vi "Detect Tags.vi"(8 "error in (no error)":errorcluster, 10 "Greyscale Image":refnum<data-value>, 11 "AprilTagDetector":refnum<data-value>) -> (0 "error out":errorcluster, 2 "Detections":T1[](array[typedef]), 3 "AprilTagDetector (Duplicate)":refnum<data-value>)   [LabVIEW 2020, in "g_ar_toolkit.feature_detection.lvlib" / "AprilTagDetector.lvclass"]
uses:
  AprilTagDetector.lvclass
  Detection.ctl
  g_ar_toolkit.common/Image Point (Float).ctl
  g_ar_toolkit.common/Square Corners.ctl
  AprilTagDetector.lvclass/AprilTagDetector.ctl
  bin/g_ar_toolkit.1.32.dll
  g_ar_toolkit.common/g_ar_toolkit.common.lvlib
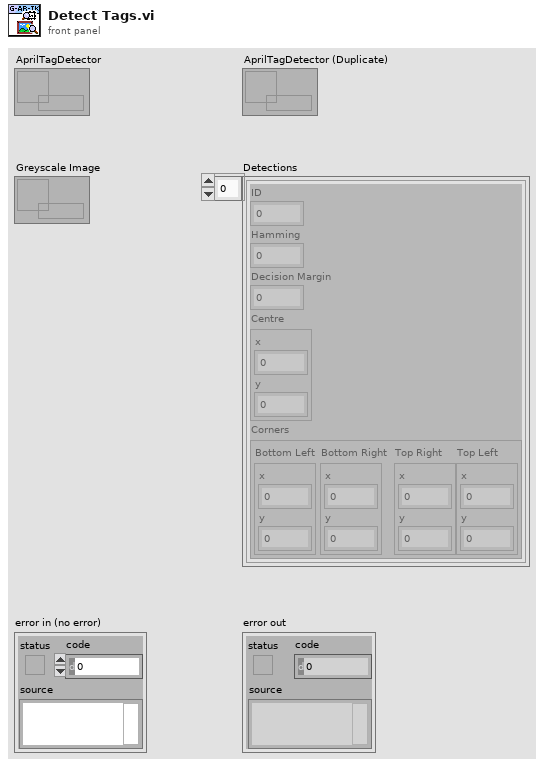
[diagram p1: front panel]
types:
  T1 = typedef "g_ar_toolkit.feature_detection.lvlib/AprilTagDetector.lvclass/Detection.ctl" = cluster{"ID":i32, "Hamming":i32, "Decision Margin":sgl, "Centre":T2, "Corners":T3}
  T2 = typedef "g_ar_toolkit.common.lvlib/Image Point (Float).ctl" = cluster{"x":dbl, "y":dbl}
  T3 = typedef "g_ar_toolkit.common.lvlib/Square Corners.ctl" = cluster{"Bottom Left":T2, "Bottom Right":T2, "Top Right":T2, "Top Left":T2}
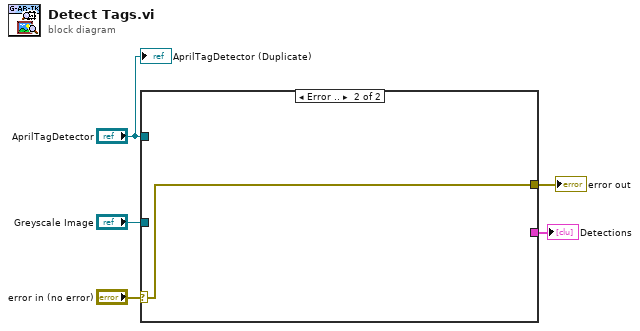
[diagram p0: block diagram]
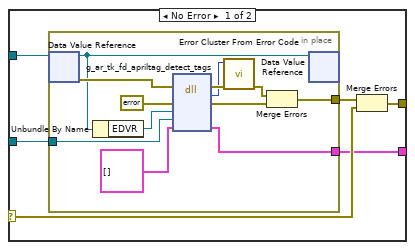
[diagram p2: hidden frame]
diagram:
  n1 = case shown="Error .." "error in (no error)" {
    selector: "error in (no error)" -> [w9 w24]
    tunnel: "Greyscale Image" -> [w11 _]
    tunnel: [w8 w24] -> w3
    tunnel: "AprilTagDetector" -> [w7 _]
    tunnel: [w6 _] -> w1
    frame No Error {
      n2 = in-place {
        in-place-border: w11 -> [w18]
        in-place-border: [w16] -> w10
        in-place-border: [w12] -> w6
        n3 = in-place-dvr #1(w7) -> (w14:refnum<class "AprilTagDetector.lvclass">, w17:errorcluster)
        n4 = Unbundle By Name(w14) -> ("EDVR"=w15:refnum<data-value>)
        n5 = dll-call lib="C:/serenial/libraries/g-augmented-reality-toolkit/LabVIEW/bin/g_ar_toolkit.1.*.*" fn="g_ar_tk_fd_apriltag_detect_tags" ("g_ar_toolkit.*.*:g_ar_tk_capture_context_create")(error in=w17, "error_cluster"=errorcluster {"status"=FALSE, "code"=0, "source"=""} ("error constant"), "Detector_EDVR"=w15, "Image_EDVR"=w18, "Detections"=T1[] [] ("Array")) -> (error out=w23:errorcluster, "MgErr"=w22:i32, "error_cluster"=w19:errorcluster, "Detections"=w12:T1[])  [unwired: 4 in, 1 out]
        n6 = call <vilib>:"Error Cluster From Error Code.vi"("error in (no error)"=w23, "error code (0)"=w22) -> ("error out"=w21:errorcluster)  [unwired: 7 in]
        n7 = Merge Errors(w21, w19) -> (w16:errorcluster)
        n8 = in-place-dvr #1(w14) -> ()  [unwired: 2 out]
      }
      n9 = Merge Errors(w10, w9) -> (w8:errorcluster)
    }
    frame Error {
    }
  }
  "error out" <- w3
  "Detections" <- w1
  "AprilTagDetector (Duplicate)" <- "AprilTagDetector"
